vi "Set ObjData.vi"(8 "error in (no error)":errorcluster, 10 "ObjData":T1, 11 "Log_Engine in":refnum<class "Log_Engine.lvclass">) -> (0 "error out":errorcluster, 3 "Log_Engine out":refnum<class "Log_Engine.lvclass">)   [LabVIEW 2019, in "Log_Engine.lvclass"]
doc: "Developed by Kevin Thompson\nkevin@thompsonengineering.net\n\nCopyright 2018\nThompson Engineering, LLC"
uses:
  Log_Engine.lvclass
  DataTypes/ObjData--cluster.ctl
  DataTypes/Read Data--cluster.ctl
  DataTypes/Settings--cluster.ctl
  Common/DataTypes/TD Async CmdMsg EventData--cluster.ctl
  DataTypes/Public Events--cluster.ctl
  DataTypes/Dependency--cluster.ctl
  Config/Config.lvclass
  DAQ_Engine/DAQ_Engine.lvclass
  Common/DataTypes/ChannelWaveforms--cluster.ctl
  Common/DataTypes/InverterWaveforms--cluster.ctl
  Common/DataTypes/InverterWaveforms--QRef.ctl
  Common/DataTypes/LogState--enum.ctl
  DataTypes/LogStateEvData--cluster.ctl
  DataTypes/LogStateChg EvData--cluster.ctl
  Common/DataTypes/TDMSState--enum.ctl
  DataTypes/TDMSStateEvData--cluster.ctl
  DataTypes/TDMSStateChg EvData--cluster.ctl
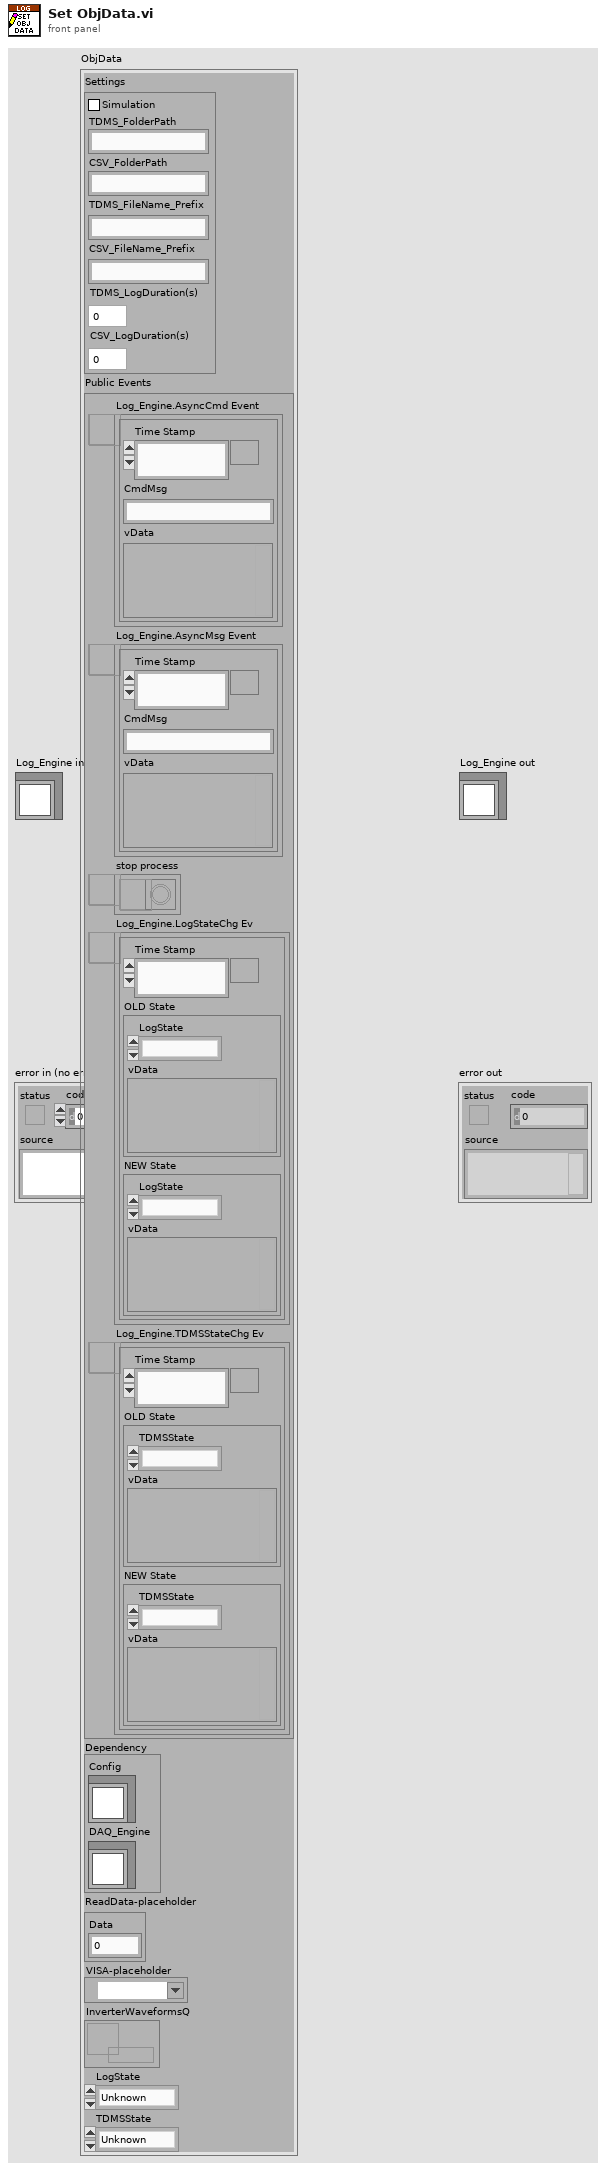
[diagram p1: front panel]
types:
  T1 = typedef "Log_Engine.lvclass/ObjData--cluster.ctl" = cluster{"Settings":T2, "Public Events":T3, "Dependency":T4, "ReadData-placeholder":T5, "VISA-placeholder":refnum<visa-resource-name>, "InverterWaveformsQ":T6, "LogState":T7, "TDMSState":T8}
  T2 = typedef "Log_Engine.lvclass/Settings--cluster.ctl" = cluster{"Simulation":bool, "TDMS_FolderPath":string, "CSV_FolderPath":string, "TDMS_FileName_Prefix":string, "CSV_FileName_Prefix":string, "TDMS_LogDuration(s)":dbl, "CSV_LogDuration(s)":dbl}
  T3 = typedef "Log_Engine.lvclass/Public Events--cluster.ctl" = cluster{"Log_Engine.AsyncCmd Event":refnum<user-event>, "Log_Engine.AsyncMsg Event":refnum<user-event>, "stop process":refnum<user-event>, "Log_Engine.LogStateChg Ev":refnum<user-event>, "Log_Engine.TDMSStateChg Ev":refnum<user-event>}
  T4 = typedef "Log_Engine.lvclass/Dependency--cluster.ctl" = cluster{"Config":refnum<class "Config.lvclass">, "DAQ_Engine":refnum<class "DAQ_Engine.lvclass">}
  T5 = typedef "Log_Engine.lvclass/Read Data--cluster.ctl" = cluster{"Data":dbl}
  T6 = typedef "InverterWaveforms--QRef.ctl" = refnum<queue>
  T7 = typedef "LogState--enum.ctl" = enum16{"Unknown", "Stopped", "Running", "Error"}
  T8 = typedef "TDMSState--enum.ctl" = enum16{"Unknown", "Stopped", "Running", "Error"}
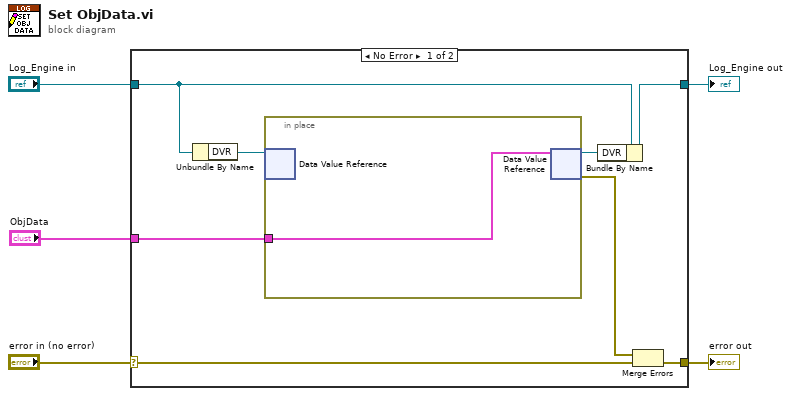
[diagram p0: block diagram]
diagram:
  n1 = case shown="No Error" "error in (no error)" {
    selector: "error in (no error)" -> [w13 w15]
    tunnel: [w7 w15] -> w4
    tunnel: [w9 w16] -> w2
    tunnel: "Log_Engine in" -> [w12 w16]
    tunnel: "ObjData" -> [w8 _]
    frame No Error {
      n2 = Unbundle By Name(w12) -> ("DVR"=w11:refnum<data-value>)
      n3 = in-place {
        in-place-border: w8 -> [w14]
        n4 = in-place-dvr #1(w11) -> ()  [unwired: 2 out]
        n5 = in-place-dvr #1(w14) -> (w10:refnum<data-value>, w6:errorcluster)
      }
      n6 = Bundle By Name(cluster=w12, "DVR"=w10) -> (w9:refnum<class "Log_Engine.lvclass">)
      n7 = Merge Errors(w6, w13) -> (w7:errorcluster)
    }
    frame Error {
    }
  }
  "error out" <- w4
  "Log_Engine out" <- w2
